vi "GetSubPanelVIName.vi"(0 "VIName":string, 5 "SubPanelLabel":string="Sub Panel", 11 "error in (no error)":errorcluster) -> (4 "VI Name":string, 15 "error out":errorcluster)   [LabVIEW 2016]
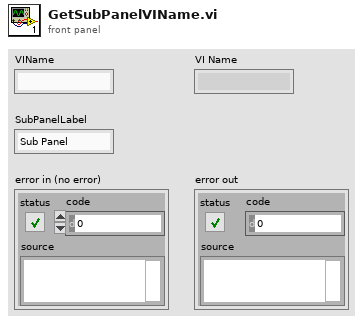
[diagram p1: front panel]
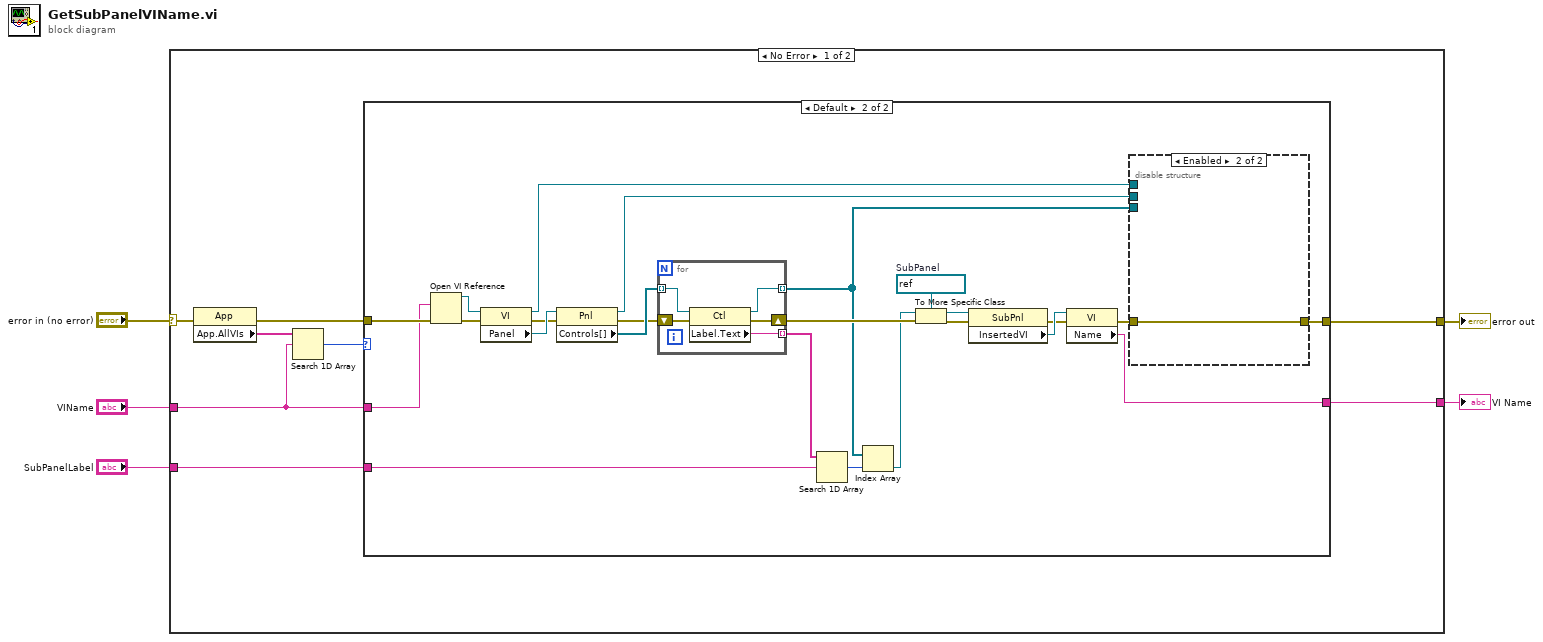
[diagram p0: block diagram]
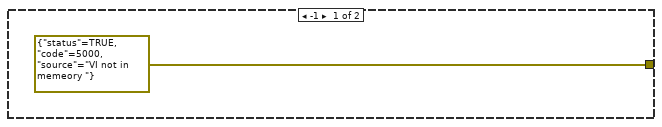
[diagram p2: hidden frame]
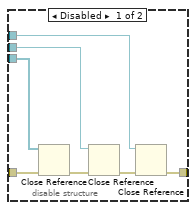
[diagram p3: hidden frame]
diagram:
  n1 = case shown="No Error" "error in (no error)" {
    selector: "error in (no error)" -> [w13 w52]
    tunnel: "VIName" -> [w7 _]
    tunnel: [w12 w52] -> w3
    tunnel: "SubPanelLabel" -> [w11 _]
    tunnel: [w10 _] -> w1
    frame No Error {
      n2 = property class="App"(error in=w13) -> (error out=w9:errorcluster, "App.AllVIs"=w8:string[])  [unwired: 1 in, 1 out]
      n3 = Search 1D Array(1D array=w8, element=w7) -> (index of element=w6:i32)  [unwired: 1 in]
      n4 = case shown="Default" w6 {
        tunnel: [errorcluster {"status"=TRUE, "code"=5000, "source"="VI not in memeory "} ("error out") w26] -> w12
        tunnel: w11 -> [_ w22]
        tunnel: [_ w18] -> w10
        tunnel: w9 -> [_ w16]
        tunnel: w7 -> [_ w15]
        frame -1 {
        }
        frame Default {
          w37 = refnum<vi> refnum  # SubPanel
          n5 = Open VI Reference(vi path=w15, error in (no error)=w16) -> (vi reference=w33:refnum<vi>, error out=w32:errorcluster)  [unwired: 4 in]
          n6 = property class="VI"(reference=w33, error in=w32) -> (reference out=w25:refnum<vi>, error out=w31:errorcluster, "Panel"=w34:refnum<vi>)
          n7 = property class="Pnl"(reference=w34, error in=w31) -> (reference out=w24:refnum<vi>, error out=w30:errorcluster, "Controls[]"=w35:refnum<vi>[])
          n8 = for {
            tunnel: w35 -> [w51] mode=indexing
            tunnel: [w50] -> w23 mode=indexing
            shift-right: [w47] -> w29
            shift-left: w30 -> [w48]
            tunnel: [w49] -> w19 mode=indexing
            n9 = property class="Ctl"(reference=w51, error in=w48) -> (reference out=w49:refnum<vi>, error out=w47:errorcluster, "Label.Text"=w50:string)
          }
          n10 = Search 1D Array(1D array=w23, element=w22) -> (index of element=w21:i32)  [unwired: 1 in]
          n11 = Index Array(array=w19, index=w21) -> (element=w20:refnum<vi>)
          n12 = To More Specific Class(target class=w37, reference=w20, error in=w29) -> (specific class reference=w36:refnum<vi>, error out=w28:errorcluster)
          n13 = property class="SubPnl"(reference=w36, error in=w28) -> (error out=w27:errorcluster, "InsertedVI"=w38:refnum<vi>)  [unwired: 1 out]
          n14 = property class="VI"(reference=w38, error in=w27) -> (error out=w17:errorcluster, "Name"=w18:string)  [unwired: 1 out]
          n15 = disable-structure shown="Enabled" {
            disable-tunnel: [w45 w46] -> w26
            disable-tunnel: w25 -> [w44 _]
            disable-tunnel: w24 -> [w43 _]
            disable-tunnel: w19 -> [w42 _]
            disable-tunnel: w17 -> [w41 w46]
            frame Disabled {
              n16 = Close Reference(reference=w42, error in (no error)=w41) -> (error out=w39:errorcluster)
              n17 = Close Reference(reference=w43, error in (no error)=w39) -> (error out=w40:errorcluster)
              n18 = Close Reference(reference=w44, error in (no error)=w40) -> (error out=w45:errorcluster)
            }
            frame Enabled {
            }
          }
        }
      }
    }
    frame Error {
    }
  }
  "error out" <- w3
  "VI Name" <- w1
